vi "Class Object Reference..FGV.vi"(6 "Connection Name":string, 7 "FGV State (GET)":T1, 8 "error in (no error)":errorcluster, 11 "LabSSH ref in":refnum<k24>) -> (0 "error out":errorcluster, 3 "LabSSH ref out":refnum<k24>)   [LabVIEW 2015, in "LabSSH.lvlib"]
doc: "<License>This software is distributed under the BSD 3-Clause License. For the full license please see license.txt or visit www.labvolution.com/license</License>"
uses:
  LabSSH.lvlib
  FGV State..enum.ctl
  C:/Working Folder/ssh.git/LabSSH Library/References/LabSSH.dll
  References/LabSSH.dll
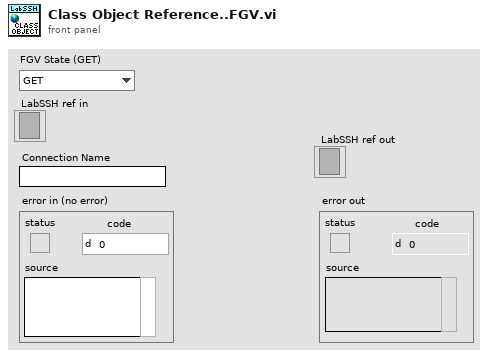
[diagram p1: front panel]
types:
  T1 = typedef "LabSSH.lvlib/FGV State..enum.ctl" = enum16{"GET", "SET"}
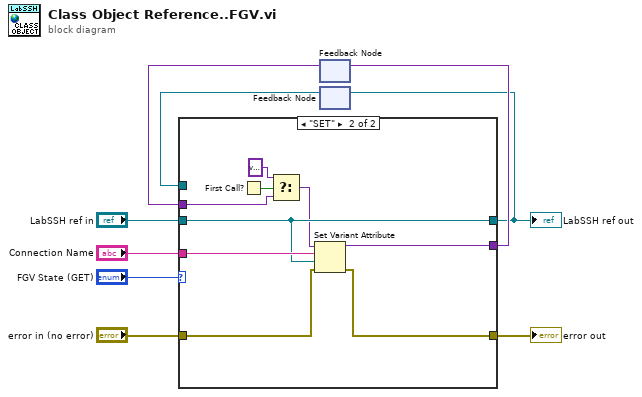
[diagram p0: block diagram]
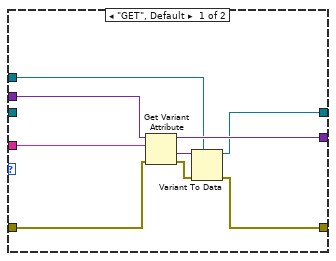
[diagram p2: hidden frame]
diagram:
  n1 = feedback #1() -> (w3:variant)  [unwired: 1 in]
  n2 = feedback #2() -> (w1:refnum<k24>)  [unwired: 1 in]
  n3 = case shown="\"SET\"" "FGV State (GET)" {
    tunnel: "error in (no error)" -> [w11 w24]
    tunnel: [w10 w23] -> w8
    tunnel: "LabSSH ref in" -> [_ w25]
    tunnel: [w13 w25] -> w2
    tunnel: "Connection Name" -> [w18 w27]
    tunnel: [w16 w26] -> w4
    tunnel: w3 -> [w17 w20]
    tunnel: w1 -> [w14 _]
    frame "GET", Default {
      n4 = Get Variant Attribute(Variant=w17, name=w18, error in=w11) -> (duplicate Variant=w16:variant, value=w15:variant, error out=w12:errorcluster)  [unwired: 1 in, 1 out]
      n5 = Variant To Data(error in=w12, type=w14, Variant=w15) -> (data=w13:refnum<k24>, error out=w10:errorcluster)
    }
    frame "SET" {
      n6 = First Call?() -> (First Call?: T/F=w21:bool)
      n7 = Select(t=variant ("variant"), s=w21, f=w20) -> (s? t:f=w19:variant)
      n8 = Set Variant Attribute(Variant=w19, name=w27, value=w25, error in=w24) -> (Variant out=w26:variant, error out=w23:errorcluster)  [unwired: 1 out]
    }
  }
  "error out" <- w8
  "LabSSH ref out" <- w2
  n9 = feedback-in #1(w4) -> ()
  n10 = feedback-in #2(w2) -> ()
